vi "test Parse File Info.vi"(11 "Test Case In":refnum<class "test Electronic Datasheet.lvclass">) -> (0 "error out":errorcluster, 3 "Test Case Out":refnum<class "test Electronic Datasheet.lvclass">)   [LabVIEW 2024, in "test Electronic Datasheet.lvclass"]
uses:
  test Electronic Datasheet.lvclass
  C:/Program Files/National Instruments/LabVIEW 2024/vi.lib/Astemes/LUnit/Test Case.lvclass
  <vilib>/PNR/JSONtext Object Serialization/Generic Object Serializer/Generic Object Serializer.lvclass
  C:/Program Files/National Instruments/LabVIEW 2024/vi.lib/JDP Science/JSONtext/LVClass Serializer/JSONtext LVClass Serializer.lvclass
  <vilib>/PNR/JSONtext Object Serialization/Generic Object Serializer/Type Name Handling.ctl
  <vilib>/PNR/JSONtext Object Serialization/Generic Object Serializer/Generic Object Serializer.lvclass/Generic Object Serializer.ctl
  <vilib>/Astemes/LUnit/Test Case.lvclass/Test Case.ctl
  e7a2ff47-5664-4bcf-a5df-3b8eb6edaa5e.vi
  4993e8ee-a06a-463a-9684-69129f64d5ce.vi
  <vilib>/PNR/JSONtext Object Serialization/Generic Object Serializer/Write Type Name Handling.vi
  <vilib>/Astemes/LUnit/Append Pass Result.vi
  <vilib>/Astemes/LUnit/Append Fail Result.vi
  <vilib>/Astemes/LUnit/Describe Comparison.vi
  4993e8ee-a06a-463a-9684-69129f64d5ce.vi/9c5d11cd-9439-4240-a1ee-d9baace9c924.vi
  <vilib>/Astemes/LUnit/Run In UI.vi
  <vilib>/Utility/error.llb/Clear Errors.vi
  Electronic Datasheet/utils/Electronic Datasheet_GetAttributes.vi
  <vilib>/JDP Science/JSONtext/Variant to JSON Text.vi
  <vilib>/Astemes/LUnit/Describe Variant.vi
  Electronic Datasheet/Electronic Datasheet.lvclass
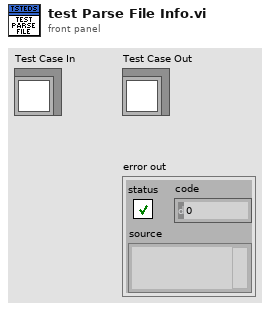
[diagram p1: front panel]
types:
  T1 = typedef "Generic Object Serializer.lvclass/Type Name Handling.ctl" = enum16{"None", "Inline"}
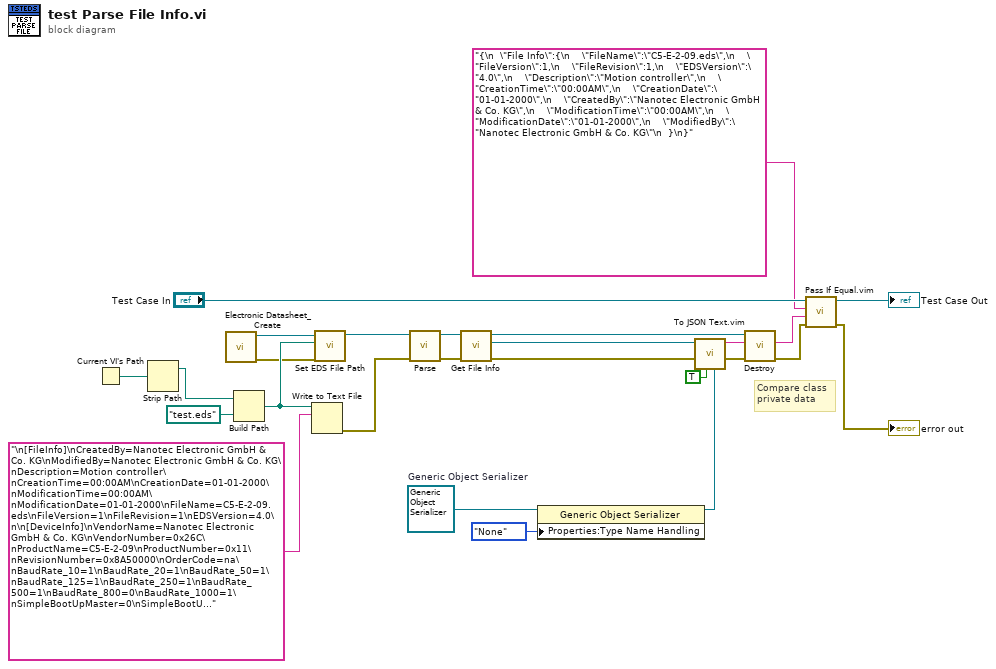
[diagram p0: block diagram]
diagram:
  w12 = refnum<class "Generic Object Serializer.lvclass"> refnum  # Generic Object Serializer
  # "Compare class\nprivate data"
  n1 = Current VI's Path() -> (path=w21:path)
  n2 = Strip Path(path=w21) -> (stripped path=w20:path)  [unwired: 1 out]
  n3 = call "Electronic Datasheet_Create.vi"() -> ("Error Out"=w3:errorcluster, "reference out"=w4:refnum<class "Electronic Datasheet.lvclass">)  [unwired: 10 in]
  n4 = Build Path(base path=w20, name or relative path=path "test.eds") -> (appended path=w19:path)
  n5 = Write to Text File(file (use dialog)=w19, text="\n[FileInfo]\nCreatedBy=Nanotec Electronic GmbH & Co. KG\nModifiedBy=Nanotec Electronic GmbH & Co. KG\nDescription=Motion controller\nCreationTime=00:00AM\nCreationDate=01-01-2000\nModificationTime=00:00AM\nModificationDate=01-01-2000\nFileName=C5-E-2-09.eds\nFileVersion=1\nFileRevision=1\nEDSVersion=4.0\n\n[DeviceInfo]\nVendorName=Nanotec Electronic GmbH & Co. KG\nVendorNumber=0x26C\nProductName=C5-E-2-09\nProductNumber=0x11\nRevisionNumber=0x8A50000\nOrderCode=na\nBaudRate_10=1\nBaudRate_20=1\nBaudRate_50=1\nBaudRate_125=1\nBaudRate_250=1\nBaudRate_500=1\nBaudRate_800=0\nBaudRate_1000=1\nSimpleBootUpMaster=0\nSimpleBootUpSlave=0\nGranularity=8\nDynamicChannelsSupported=0\nCompactPDO=0\nGroupMessaging=0\nNrOfRXPDO=8\nNrOfTXPDO=8\nLSS_Supported=0\n") -> (error out=w17:errorcluster)  [unwired: 2 in, 2 out]
  n6 = call "Set EDS File Path.vi"("error in"=w3, "EDS File Path"=w19, "reference in"=w4) -> ("reference out"=w22:refnum<class "Electronic Datasheet.lvclass">)  [unwired: 7 in, 1 out]
  n7 = call "Parse.vi"("error in"=w17, "reference in"=w22) -> ("error out"=w8:errorcluster, "reference out"=w15:refnum<class "Electronic Datasheet.lvclass">)  [unwired: 8 in]
  n8 = call "Get File Info.vi"("reference in"=w15) -> ("File Info"=w6:refnum<class "File Info.lvclass">, "reference out"=w1:refnum<class "Electronic Datasheet.lvclass">)  [unwired: 9 in]
  n9 = property class="Generic Object Serializer"(reference=w12, "Properties:Type Name Handling"=Type_Name_Handling."None" ("Type Name Handling")) -> (reference out=w11:refnum<class "Generic Object Serializer.lvclass">)  [unwired: 1 in, 1 out]
  n10 = call "To JSON Text.vim"("LVClass Serializer"=w11, "Pretty Print?"=TRUE, "error in (no error)"=w8, "Anything"=w6) -> ("error out"=w5:errorcluster, "<JSON>"=w7:string)  [unwired: 6 in]
  n11 = call-dynamic "Destroy.vi"("Error In"=w5, "reference in"=w1) -> ("Error Out"=w2:errorcluster)  [unwired: 8 in, 1 out]
  n12 = call "Pass If Equal.vim"("error in (no error)"=w2, "Actual"=w7, "Expected"="{\n  \"File Info\":{\n    \"FileName\":\"C5-E-2-09.eds\",\n    \"FileVersion\":1,\n    \"FileRevision\":1,\n    \"EDSVersion\":\"4.0\",\n    \"Description\":\"Motion controller\",\n    \"CreationTime\":\"00:00AM\",\n    \"CreationDate\":\"01-01-2000\",\n    \"CreatedBy\":\"Nanotec Electronic GmbH & Co. KG\",\n    \"ModificationTime\":\"00:00AM\",\n    \"ModificationDate\":\"01-01-2000\",\n    \"ModifiedBy\":\"Nanotec Electronic GmbH & Co. KG\"\n  }\n}" ("<JSON>"), "LUnit Test Case In"="Test Case In") -> ("error out"=→"error out":errorcluster, "LUnit Test Case Out"=→"Test Case Out":refnum<class "test Electronic Datasheet.lvclass">)  [unwired: 6 in]
